vi "Periodic Tasks.vi"(8 "error in":errorcluster) -> ()   [LabVIEW 2013]
doc: "This VI runs in parallel to other tasks. It can contain as many user-defined periodic loops as you need. These can carry out PID or other sorts of timed response."
uses:
  <vilib>/Rock Robotics/SystemInterfaces/DIO/FPGA_DIOChannel.ctl
  <vilib>/Rock Robotics/SystemInterfaces/Utilities/FPGA_UtilitiesLED Source.ctl
  <vilib>/Rock Robotics/SystemInterfaces/Utilities/FPGA_UtilitiesLED State.ctl
  Program Files/National Instruments/LabVIEW 2013/examples/FRC/I2C/ADXL345 I2C/Driver/ADXL345 I2C Axis.ctl
  <vilib>/Analysis/baseanly.llb/Mean (DBL).vi
  Robot Global Data.vi
  <vilib>/Rock Robotics/WPI/Compressor/WPI_CompressorGetSetRefNum.vi
  <vilib>/Rock Robotics/WPI/RobotDrive/WPI_RobotDriveGetSetRefNum.vi
  <vilib>/Rock Robotics/WPI/Joystick/WPI_JoystickGetSetRefNum.vi
  Vision Data.vi
  Encoder Data.vi
  Angle.vi
  <vilib>/Analysis/NI_AALBase.lvlib
panel:
  out "Average Distance":dbl format="%0.2f"
  out "Hall Effect Sensor":bool
  out "Acceleration (m/s^2)":dbl
  out "Acceleration (G)":dbl
  out "Angle (for Gyro)":dbl
  out "Left Rotation":dbl
  out "Right Rotation":dbl
  out "Left Distance":dbl
  out "Right Distance":dbl
  out "Cam Distance (in)":dbl
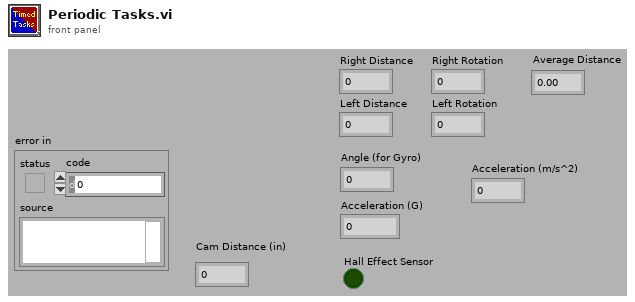
[diagram p1: front panel]
types:
  T1 = typedef "FPGA_DIOChannel.ctl" = enum8{"DIO 1", "DIO 2", "DIO 3", "DIO 4", "DIO 5", "DIO 6", "DIO 7", "DIO 8", "DIO 9", "DIO 10", "DIO 11", "DIO 12", "DIO 13", "DIO 14", "Invalid"}
  T2 = typedef "ADXL345 I2C Axis.ctl" = u8
  T3 = typedef "WPI_I2CDevRef.ctl" = cluster{"DevStatus":errorcluster, "Digital Module":T4, "Device Address":u8}
  T4 = typedef "FPGA_TypedefDigitalModule.ctl" = enum16{"Digital Module 1", "Digital Module 2"}
  T5 = typedef "WPI_DigitalInputDevRef.ctl" = cluster{"DevStatus":errorcluster, "DIO Channel":T1, "Digital Module":T4}
  T6 = typedef "WPI_GyroDevRef.ctl" = cluster{"DevStatus":errorcluster, "Analog Module":T7, "Analog Channel":T8, "Offset":dbl, "Gain (VoltsPerDegree/Second)":dbl}
  T7 = typedef "FPGA_TypedefAnalogModule.ctl" = enum16{"Analog Module 1", "Analog Module 2"}
  T8 = typedef "FPGA_AIChannel.ctl" = enum8{"AI 1", "AI 2", "AI 3", "AI 4", "AI 5", "AI 6", "AI 7", "AI 8", "Invalid"}
  T9 = typedef "WPI_JoystickDevRef.ctl" = cluster{"Device":T10}
  T10 = typedef "WPI_JoystickDeviceEnum.ctl" = enum16{"USB 1", "USB 2", "USB 3", "USB 4", "Kinect 1", "Kinect 2"}
  T11 = typedef "WPI_RobotDriveDevRef.ctl" = cluster{"DevStatus":errorcluster, "Motors[]":T12[], "Square Inputs":bool, "Max Output":dbl, "Isochronous":bool}
  T12 = typedef "WPI_MotorControlDeviceRef.ctl" = cluster{"DeviceStatus":errorcluster, "Type":enum16{"PWM", "CAN"}, "PWM":cluster{"Digital Module":T4, "PWM Channel":T13, "DeadBand":T14}, "CAN":cluster{"Device Number":u8, "Control Mode":T15, "Semaphore":T16, "Max Vout":dbl}, "Invert":bool, "TransformRef":T17, "InvTransformRef":T17}
  T13 = typedef "FPGA_DIOPWMChannel.ctl" = enum8{"PWM 1", "PWM 2", "PWM 3", "PWM 4", "PWM 5", "PWM 6", "PWM 7", "PWM 8", "PWM 9", "PWM 10", "Invalid"}
  T14 = typedef "WPI_PWMDeadband.ctl" = cluster{"Name":string, "maxPositivePwm":i32, "minPositivePwm":i32, "centerPwm":i32, "maxNegativePwm":i32, "minNegativePwm":i32, "angularRange":u16}
  T15 = typedef "WPI_CANJaguar_ControlMode.ctl" = enum8{"Percent VBus", "Current", "Speed", "Position", "Voltage"}
  T16 = typedef "Semaphore RefNum" = refnum<k1>
  T17 = typedef "WPI_PWMTransform_ConPane.ctl" = refnum<vi>
  T18 = typedef "WPI_CompressorDevRef.ctl" = cluster{"DevStatus":errorcluster, "DigitalInputDevRef":T5, "RelayDevRef":T19}
  T19 = typedef "WPI_RelayDevRef.ctl" = cluster{"DevStatus":errorcluster, "Relay Channel":T20, "Digital Module":T4, "Relay Direction":T21}
  T20 = typedef "FPGA_DIORelayChannel.ctl" = enum8{"Relay 1", "Relay 2", "Relay 3", "Relay 4", "Relay 5", "Relay 6", "Relay 7", "Relay 8", "Invalid"}
  T21 = typedef "WPI_RelayDirection.ctl" = enum16{"Both directions", "Forward only", "Reverse only"}
  T22 = typedef "WPI_EncoderDevRef.ctl" = cluster{"DevStatus":errorcluster, "EncoderIndex":T23, "CounterIndex":T24, "DistancePerCount":dbl, "Decoding Type":T25}
  T23 = typedef "FPGA_EncoderIdx.ctl" = enum8{"Enc 0", "Enc 1", "Enc 2", "Enc 3", "Invalid"}
  T24 = typedef "FPGA_CounterCtrSystemIndex.ctl" = enum8{"Ctr 0", "Ctr 1", "Ctr 2", "Ctr 3", "Ctr 4", "Ctr 5", "Ctr 6", "Ctr 7", "Invalid"}
  T25 = typedef "WPI_EncoderType.ctl" = enum16{"1x", "2x", "4x"}
  T26 = cluster{"JoystickDevRef":T9, "RobotDriveDevRef":T11}
  T27 = typedef "FPGA_UtilitiesLED State.ctl" = enum16{"Off", "On", "Toggle"}
  T28 = typedef "FPGA_UtilitiesLED Source.ctl" = enum16{"User LED", "FPGA LED"}
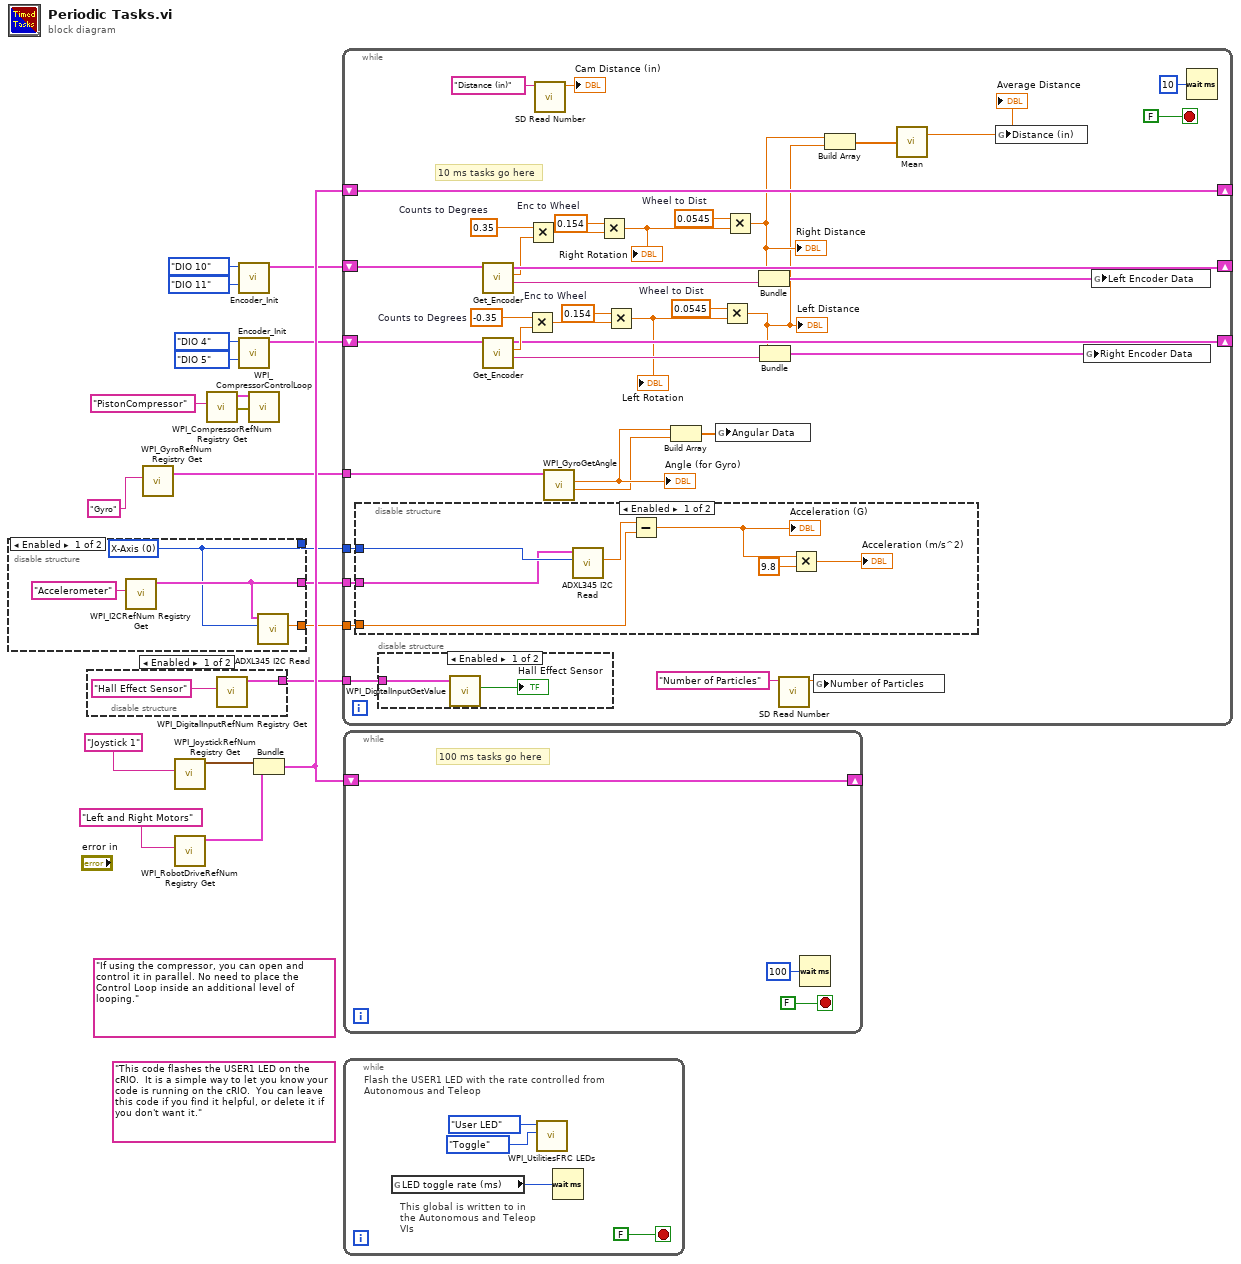
[diagram p0: block diagram]
diagram:
  (unwired) "If using the compressor, you can open and control it in parallel. No need to place the Control Loop inside an additional level of looping."
  (unwired) "This code flashes the USER1 LED on the cRIO.  It is a simple way to let you know your code is running on the cRIO.  You can leave this code if you find it helpful, or delete it if you don't want it."
  n1 = disable-structure shown="Enabled" {
    disable-tunnel: [w23 _] -> w4
    disable-tunnel: [w22 _] -> w3
    disable-tunnel: [w21 _] -> w2
    frame Enabled {
      w22 = T2 0 items=["X-Axis", "Y-Axis", "Z-Axis"] ("Axis")
      n2 = call <vilib>:"WPI_I2CRefNum Registry Get.vi"("refnum name"="Accelerometer") -> ("I2CDevRef"=w23:T3)  [unwired: 9 in, 1 out]
      n3 = call "ADXL345 I2C Read.vi"("Axis"=w22, "I2CDevRef"=w23) -> ("Acceleration"=w21:dbl)  [unwired: 1 in, 8 out]
    }
    frame Disabled {
    }
  }
  n4 = disable-structure shown="Enabled" {
    disable-tunnel: [w25 _] -> w1
    frame Enabled {
      n5 = call <vilib>:"WPI_DigitalInputRefNum Registry Get.vi"("refnum name"="Hall Effect Sensor") -> ("DigitalInputDevRef"=w25:T5)  [unwired: 9 in, 1 out]
    }
    frame Disabled {
    }
  }
  n6 = call <vilib>:"WPI_GyroRefNum Registry Get.vi"("refnum name"="Gyro") -> ("GyroDevRef"=w5:T6)  [unwired: 9 in, 1 out]
  n7 = call <vilib>:"WPI_JoystickRefNum Registry Get.vi"("refnum name"="Joystick 1") -> ("JoystickDevRef"=w18:T9)  [unwired: 1 in, 9 out]
  n8 = call <vilib>:"WPI_RobotDriveRefNum Registry Get.vi"("refnum name"="Left and Right Motors") -> ("RobotDriveDevRef"=w17:T11)  [unwired: 1 in, 9 out]
  n9 = call <vilib>:"WPI_CompressorRefNum Registry Get.vi"("refnum name"="PistonCompressor") -> ("error out"=w7:errorcluster, "CompressorDevRef"=w8:T18)  [unwired: 9 in]
  n10 = call "Encoder_Init.vi"("B Channel"=FPGA_DIOChannel."DIO 11", "A Channel"=FPGA_DIOChannel."DIO 10") -> ("EncoderDevRef"=w15:T22)  [unwired: 9 in]
  n11 = call "Encoder_Init.vi"("B Channel"=FPGA_DIOChannel."DIO 5", "A Channel"=FPGA_DIOChannel."DIO 4") -> ("EncoderDevRef"=w10:T22)  [unwired: 9 in]
  n12 = call <vilib>:"WPI_CompressorControlLoop.vi"("error in (no error)"=w7, "CompressorDevRef"=w8) -> ()  [unwired: 10 in]
  n13 = Bundle("JoystickDevRef"=w18, "RobotDriveDevRef"=w17) -> (w16:T26)  [unwired: 1 out]
  n14 = while {
    shift-right: [w63] -> _
    shift-left: w16 -> [w63]
    shift-right: [w61] -> _
    shift-left: w15 -> [w62]
    shift-right: [w48] -> _
    shift-left: w10 -> [w55]
    tunnel: w3 -> [w40]
    tunnel: w5 -> [w39]
    tunnel: w4 -> [w38]
    tunnel: w2 -> [w37]
    tunnel: w1 -> [w33]
    stop <- FALSE stop-if-true
    w44 = 0.0545  # Wheel to Dist
    w45 = 0.154  # Enc to Wheel
    w50 = 0.0545  # Wheel to Dist
    w51 = 0.154  # Enc to Wheel
    w58 = -0.35  # Counts to Degrees
    w59 = 0.35  # Counts to Degrees
    # "10 ms tasks go here"
    n15 = disable-structure shown="Enabled" {
      disable-tunnel: w40 -> [w74 _]
      disable-tunnel: w38 -> [w73 _]
      disable-tunnel: w37 -> [w70 _]
      frame Enabled {
        n16 = call "ADXL345 I2C Read.vi"("Axis"=w74, "I2CDevRef"=w73) -> ("Acceleration"=w71:dbl)  [unwired: 1 in, 8 out]
        n17 = Subtract(x=w71, y=w70) -> (x-y=w69:dbl)
        "Acceleration (G)" <- w69
        n18 = Multiply(x=w69, y=9.8) -> (x*y=→"Acceleration (m/s^2)":dbl)
      }
      frame Disabled {
      }
    }
    n19 = disable-structure shown="Enabled" {
      disable-tunnel: w33 -> [w67 _]
      frame Enabled {
        n20 = call <vilib>:"WPI_DigitalInputGetValue.vi"("DigitalInputDevRef"=w67) -> ("Value"=→"Hall Effect Sensor":bool)  [unwired: 8 in, 2 out]
      }
      frame Disabled {
      }
    }
    n21 = call "Get_Encoder.vi"("EncoderDevRef"=w62) -> ("Encoder Direction"=w47:string, "Encoder Distance"=w60:dbl, "EncoderDevRef 2"=w61:T22)  [unwired: 7 in, 1 out]
    n22 = call "Get_Encoder.vi"("EncoderDevRef"=w55) -> ("Encoder Direction"=w56:string, "Encoder Distance"=w57:dbl, "EncoderDevRef 2"=w48:T22)  [unwired: 7 in, 1 out]
    n23 = Multiply(x=w58, y=w57) -> (x*y=w42:dbl)
    n24 = Multiply(x=w59, y=w60) -> (x*y=w52:dbl)
    n25 = call <vilib>:"SD Read Number.vi"("Name"="Distance (in)") -> ("Numeric"=→"Cam Distance (in)":dbl)  [unwired: 8 in, 2 out]
    n26 = call <vilib>:"WPI_GyroGetAngle.vi"("GyroDevRef"=w39) -> ("Angular Rate"=w35:dbl, "Angle"=w36:dbl)  [unwired: 7 in, 2 out]
    "Angle (for Gyro)" <- w36
    n27 = Multiply(x=w51, y=w52) -> (x*y=w49:dbl)
    "Right Rotation" <- w49
    n28 = Multiply(x=w45, y=w42) -> (x*y=w43:dbl)
    "Left Rotation" <- w43
    n29 = Build Array(w36, w35) -> (w34:dbl[])
    n30 = global write "Angle.vi" "Angular Data"(w34) -> ()
    n31 = Multiply(x=w44, y=w43) -> (x*y=w30:dbl)
    "Left Distance" <- w30
    n32 = Multiply(x=w50, y=w49) -> (x*y=w31:dbl)
    "Right Distance" <- w31
    n33 = Bundle(w31, "Encoder Direction"=w47) -> (w41:cluster{dbl, "Encoder Direction":string})  [unwired: 1 in]
    n34 = Bundle(w30, "Encoder Direction"=w56) -> (w46:cluster{dbl, "Encoder Direction":string})  [unwired: 1 in]
    n35 = call <vilib>:"SD Read Number.vi"("Name"="Number of Particles") -> ("Numeric"=w27:dbl)  [unwired: 8 in, 2 out]
    n36 = global write "Vision Data.vi" "Number of Particles"(w27) -> ()
    n37 = Build Array(w31, w30) -> (w32:dbl[])
    n38 = call-poly <vilib>:"Mean.vi"("X"=w32) -> ("mean"=w29:dbl)  [unwired: 1 out]
    "Average Distance" <- w29
    n39 = global write "Vision Data.vi" "Distance (in)"(w29) -> ()
    n40 = global write "Encoder Data.vi" "Right Encoder Data"(w46) -> ()
    n41 = global write "Encoder Data.vi" "Left Encoder Data"(w41) -> ()
    n42 = Wait (ms)(milliseconds to wait=u32 10) -> ()  [unwired: 1 out]
  }
  n43 = while {
    shift-right: [w75] -> _
    shift-left: w16 -> [w75]
    stop <- FALSE stop-if-true
    # "100 ms tasks go here"
    n44 = Wait (ms)(milliseconds to wait=u32 100) -> ()  [unwired: 1 out]
  }
  n45 = while {
    stop <- FALSE stop-if-true
    # "This global is written to in the Autonomous and Teleop VIs"
    # "Flash the USER1 LED with the rate controlled from Autonomous and Teleop"
    n46 = global read "Robot Global Data.vi" "LED toggle rate (ms)"() -> (w78:u32)
    n47 = call <vilib>:"WPI_UtilitiesFRC LEDs.vi"("State"=FPGA_UtilitiesLED_State."Toggle", "LED Type"=FPGA_UtilitiesLED_Source."User LED") -> ()  [unwired: 1 in, 9 out]
    n48 = Wait (ms)(milliseconds to wait=w78) -> ()  [unwired: 1 out]
  }
